vi "Virtual Launch.vi"(8 "error in (no error)":errorcluster caption="entrée d'erreur (pas d'erreur)") -> (0 "error out":errorcluster caption="sortie d'erreur")   [LabVIEW 2020, in "Library Instrument & Equipement.lvlib" / "Process (Default).lvclass"]
uses:
  Process (Default).lvclass
  Variable dispatch.vi
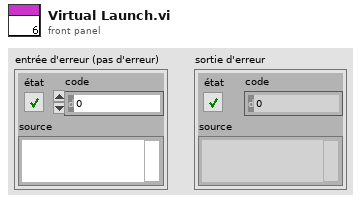
[diagram p1: front panel]
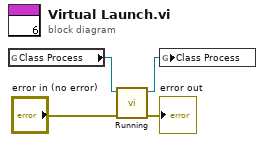
[diagram p0: block diagram]
diagram:
  n1 = global read "Variable dispatch.vi" "Class Process"() -> (w2:refnum<class "Process (Default).lvclass">)
  n2 = call-dynamic "Running.vi"("error in (no error)"="error in (no error)", "Process (Default) en entrée"=w2) -> ("error out"=→"error out":errorcluster, "Process (Default) en sortie"=w1:refnum<class "Process (Default).lvclass">)  [unwired: 8 in]
  n3 = global write "Variable dispatch.vi" "Class Process"(w1) -> ()
